vi "tempAcquisition.vi"(8 "Error IN":errorcluster caption="entrée d'erreur (pas d'erreur)", 9 "Acquisition Period":u32=100, 10 "queue IN":refnum<queue>, 11 "VISA":refnum<visa-resource-name>) -> (0 "Error OUT":errorcluster caption="sortie d'erreur")   [LabVIEW 2020]
uses:
  var globales/closeThreads.vi
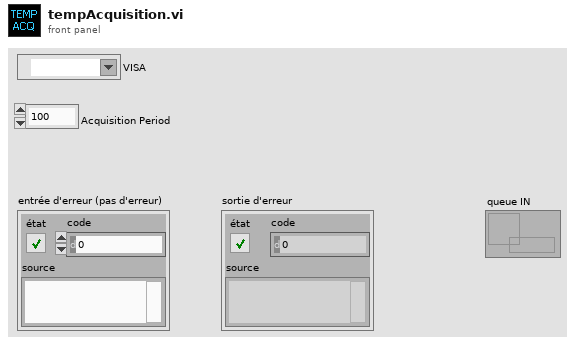
[diagram p1: front panel]
types:
  T1 = cluster{"sensor Luxtron1":dbl, "sensor Luxtron2":dbl, "sensor DAQ1":dbl, "sensor DAQ2":dbl, "temps":dbl}
  T2 = cluster{"Status_1":bool, "Value_1":dbl, "Unit_1":string, "Status_2":bool, "Value_2":dbl, "Unit_2":string, "Status_3":bool, "Value_3":dbl, "Unit_3":string, "Status_4":bool, "Value_4":dbl, "Unit_4":string}
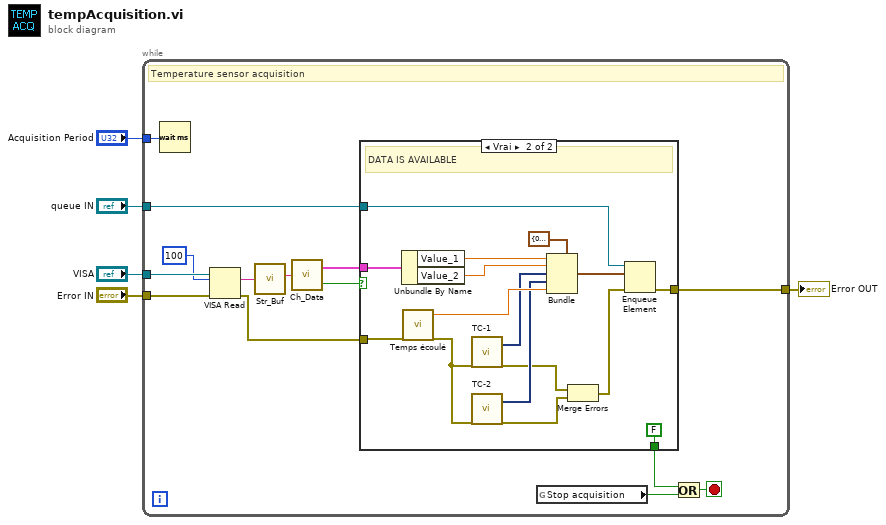
[diagram p0: block diagram]
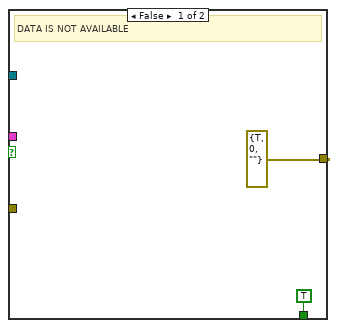
[diagram p2: hidden frame]
diagram:
  n1 = while {
    tunnel: "VISA" -> [w15]
    tunnel: "Error IN" -> [w14]
    tunnel: [w12] -> w2
    tunnel: "queue IN" -> [w16]
    tunnel: "Acquisition Period" -> [w13]
    stop <- w7 stop-if-true
    # "Temperature sensor acquisition"
    n2 = Wait (ms)(milliseconds to wait=w13) -> ()  [unwired: 1 out]
    n3 = VISA Read(VISA resource name=w15, byte count=u32 100 ("nombre d'octets"), error in (no error)=w14) -> (read buffer=w18:string, error out=w11:errorcluster)  [unwired: 2 out]
    n4 = call "Str_Buf.vi"("String_in"=w18) -> ("String_Out"=w19:string)  [unwired: 3 out]
    n5 = call "Ch_Data.vi"("String"=w19) -> ("output cluster"=w17:T2, "FormatOK"=w10:bool)
    n6 = case shown="Vrai" w10 {
      tunnel: w17 -> [_ w36]
      tunnel: w11 -> [_ w37]
      tunnel: w16 -> [_ w23]
      tunnel: [errorcluster {"status"=TRUE, "code"=0, "source"=""} ("error out") w33] -> w12
      tunnel: [TRUE FALSE] -> w8
      frame False {
        # "DATA IS NOT AVAILABLE"
      }
      frame True {
        # "DATA IS AVAILABLE"
        n7 = Unbundle By Name(w36) -> ("Value_1"=w35:dbl, "Value_2"=w34:dbl)
        n8 = call "Temps écoulé"("error in (no error)"=w37) -> ("Elapsed Time (s)"=w32:dbl, "error out"=w29:errorcluster)  [unwired: 11 in, 6 out]
        n9 = call "TC-1"("error in"=w29) -> ("data"=w31:dynamicdata, "error out"=w27:errorcluster)  [unwired: 16 in, 1 out]
        n10 = call "TC-2"("error in"=w29) -> ("data"=w30:dynamicdata, "error out"=w26:errorcluster)  [unwired: 16 in, 1 out]
        n11 = Bundle(cluster=T1 {"sensor Luxtron1"=0.0, "sensor Luxtron2"=36.42, "sensor DAQ1"=0.0, "sensor DAQ2"=0.0, "temps"=122.90212535858154} ("Temperature datas"), "sensor Luxtron1"=w35, "sensor Luxtron2"=w34, "sensor DAQ1"=w31, "sensor DAQ2"=w30, "temps"=w32) -> (w25:T1)
        n12 = Merge Errors(w27, w26) -> (w28:errorcluster)
        n13 = Enqueue Element(queue=w23, element=w25, error in (no error)=w28) -> (error out=w33:errorcluster)  [unwired: 1 in, 2 out]
      }
    }
    n14 = global read "closeThreads.vi" "Stop acquisition"() -> (w6:bool)
    n15 = Or(x=w8, y=w6) -> (x .or. y?=w7:bool)
  }
  "Error OUT" <- w2
